vi "Extract CMD_Data.vi"(11 "Frame":string) -> (0 "Frame Type":string, 1 "DATA":string, 2 "Command ID":string, 3 "Command Type":string)   [LabVIEW 2020, in "Library Test.lvlib" / "Nodon_Send_Command_UART.lvclass"]
uses:
  Nodon_Send_Command_UART.lvclass
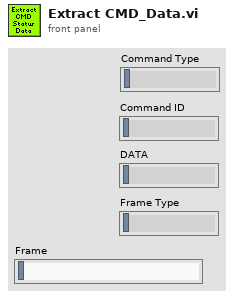
[diagram p1: front panel]
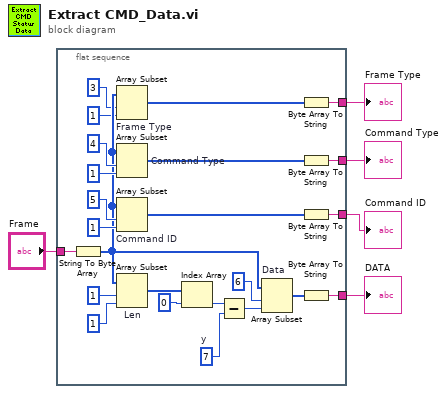
[diagram p0: block diagram]
diagram:
  n1 = flat-sequence {
    tunnel: "Frame" -> [w15]
    tunnel: [w14] -> w5
    tunnel: [w13] -> w4
    tunnel: [w11] -> w2
    tunnel: [w6] -> w1
    frame #0 {
      w19 = u8 7  # y
      n2 = String To Byte Array(string=w15) -> (unsigned byte array=w10:u8[])
      n3 = Array Subset "Frame Type"(array=w10, index=3 ("indice"), length=1 ("longueur")) -> (w7:u8[])
      n4 = Array Subset "Command Type"(array=w10, index=4 ("indice"), length=1 ("longueur")) -> (w18:u8[])
      n5 = Array Subset "Command ID"(array=w10, index=5 ("indice"), length=1 ("longueur")) -> (w12:u8[])
      n6 = Array Subset "Len"(array=w10, index=1 ("indice"), length=1 ("longueur")) -> (w28:u8[])
      n7 = Index Array(array=w28, index=0 ("indice")) -> (element=w29:u8)
      n8 = Subtract(x=w29, y=w19) -> (x-y=w17:u8)
      n9 = Array Subset "Data"(array=w10, index=6 ("indice"), length=w17) -> (w16:u8[])
      n10 = Byte Array To String(unsigned byte array=w7) -> (string=w6:string)
      n11 = Byte Array To String(unsigned byte array=w18) -> (string=w13:string)
      n12 = Byte Array To String(unsigned byte array=w12) -> (string=w11:string)
      n13 = Byte Array To String(unsigned byte array=w16) -> (string=w14:string)
    }
  }
  "DATA" <- w5
  "Command Type" <- w4
  "Command ID" <- w2
  "Frame Type" <- w1
